vi "Statistics.vi"(0 "image in":refnum<class "MSC Image.lvclass">, 1 "mask image in":refnum<class "MSC Image.lvclass">, 5 "error in (no error)":errorcluster) -> (8 "mean":dbl, 10 "stdDev":dbl, 12 "area":dbl, 14 "image out":refnum<class "MSC Image.lvclass">, 15 "mask image out":refnum<class "MSC Image.lvclass">, 16 "min":dbl, 17 "max":dbl, 19 "error out":errorcluster)   [LabVIEW 2016, in "MSC Image.lvclass"]
doc: "Calculates statistical values of an image with optional mask.\n\nThe image type double can lead to overflows."
uses:
  MSC Image.lvclass
  Dependencies/x86/MSC I Process32.dll
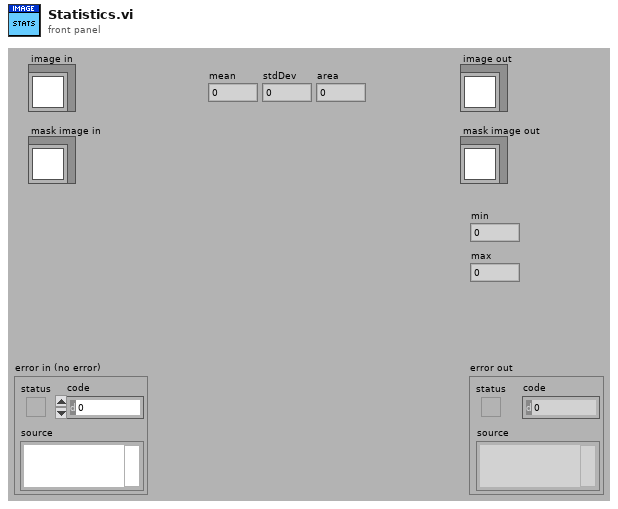
[diagram p1: front panel]
types:
  T1 = typedef "Image.ctl" = cluster{"Pointer":u64, "Size":T2, "Image Type":T3, "Time Stamp":timestamp, "Variant":variant}
  T2 = typedef "Size.ctl" = cluster{"Cols":i32, "Rows":i32}
  T3 = typedef "Image Type.ctl" = i32
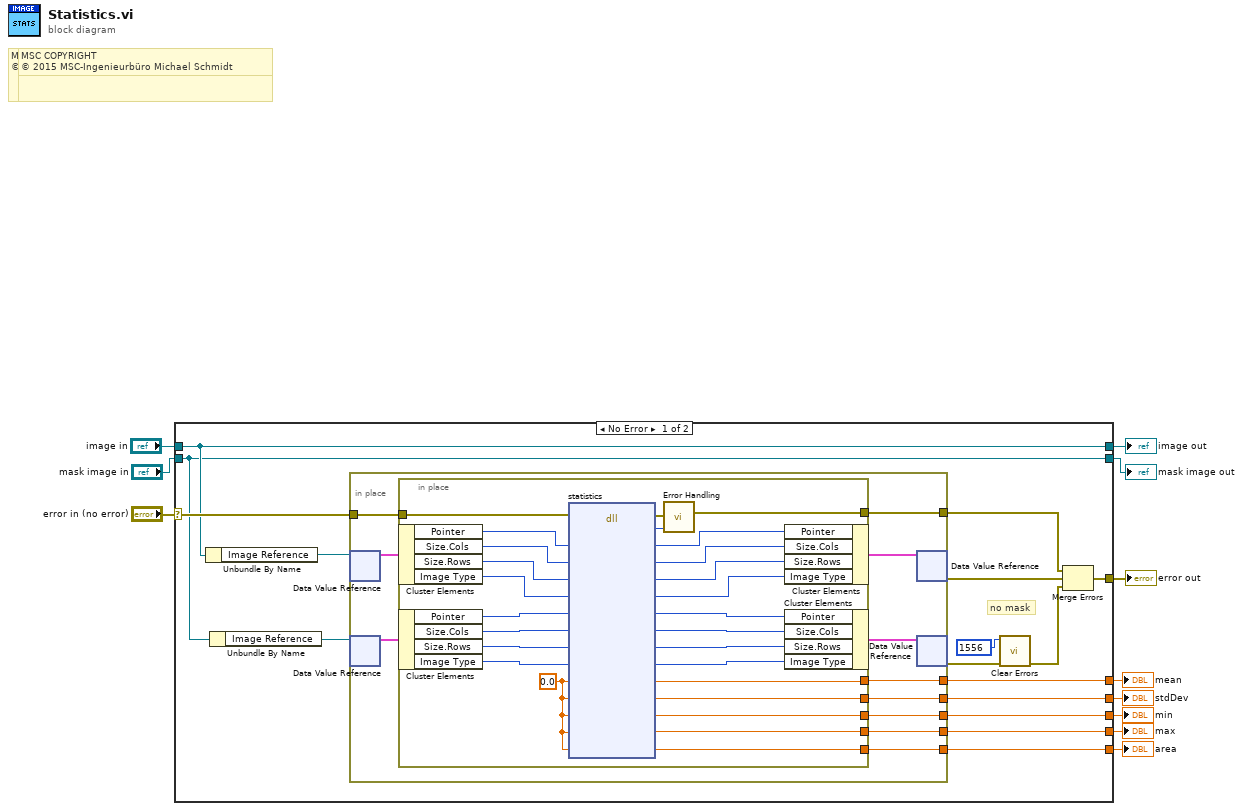
[diagram p0: block diagram]
diagram:
  # "MSC COPYRIGHT\n© 2016 MSC-Ingenieurbüro Michael Schmidt"
  # "MSC COPYRIGHT\n© 2016 MSC-Ingenieurbüro Michael Schmidt"
  # "MSC COPYRIGHT\n© 2015 MSC-Ingenieurbüro Michael Schmidt"
  # "MSC COPYRIGHT\n© 2015 MSC-Ingenieurbüro Michael Schmidt"
  n1 = case shown="No Error" "error in (no error)" {
    selector: "error in (no error)" -> [w16 w67]
    tunnel: [w27 w67] -> w6
    tunnel: [w12 w65] -> w8
    tunnel: "image in" -> [w15 w66]
    tunnel: "mask image in" -> [w12 w65]
    tunnel: [w15 w66] -> w11
    tunnel: [w21 _] -> w5
    tunnel: [w20 _] -> w4
    tunnel: [w24 _] -> w3
    tunnel: [w23 _] -> w2
    tunnel: [w22 _] -> w1
    frame No Error {
      # "no mask"
      n2 = Unbundle By Name(w15) -> ("Image Reference"=w14:refnum<data-value>)
      n3 = Unbundle By Name(w12) -> ("Image Reference"=w13:refnum<data-value>)
      n4 = in-place {
        in-place-border: w16 -> [w36]
        in-place-border: [w35] -> w26
        in-place-border: [w32] -> w21
        in-place-border: [w31] -> w20
        in-place-border: [w30] -> w24
        in-place-border: [w29] -> w23
        in-place-border: [w28] -> w22
        n5 = in-place-dvr #1(w14) -> (w37:T1)  [unwired: 1 out]
        n6 = in-place-dvr #2(w13) -> (w34:T1)  [unwired: 1 out]
        n7 = in-place {
          in-place-border: w36 -> [w39]
          in-place-border: [w50] -> w35
          in-place-border: [w64] -> w32
          in-place-border: [w63] -> w31
          in-place-border: [w62] -> w30
          in-place-border: [w61] -> w29
          in-place-border: [w60] -> w28
          w48 = 0.0 ("mean")
          n8 = in-place-cluster #3(w37) -> ("Pointer"=w47:u64, "Size.Cols"=w46:i32, "Size.Rows"=w45:i32, "Image Type"=w44:T3)
          n9 = in-place-cluster #4(w34) -> ("Pointer"=w43:u64, "Size.Cols"=w42:i32, "Size.Rows"=w41:i32, "Image Type"=w40:T3)
          n10 = dll-call lib="C:/Users/MSC/LabVIEW Projekte/LV 2014/MSC I-Process/user.lib/MSC-I Process/Dependencies/x86/MSC I Process*.dll" fn="statistics"(error in=w39, "pointer"=w47, "cols"=w46, "rows"=w45, "type"=w44, "pointerMask"=w43, "colsMask"=w42, "rowsMask"=w41, "typeMask"=w40, "mean"=w48, "stdDev"=w48, "min"=w48, "max"=w48, "area"=w48) -> (error out=w52:errorcluster, "error"=w51:i32, "pointer"=w49:u64, "cols"=w53:i32, "rows"=w54:i32, "type"=w55:i32, "pointerMask"=w59:u64, "colsMask"=w58:i32, "rowsMask"=w57:i32, "typeMask"=w56:i32, "mean"=w64:dbl, "stdDev"=w63:dbl, "min"=w62:dbl, "max"=w61:dbl, "area"=w60:dbl)  [unwired: 2 in, 1 out]
          n11 = call "Error Handling.vi"("error in (no error)"=w52, "return type"=w51) -> ("error out"=w50:errorcluster)  [unwired: 12 in, 1 out]
          n12 = in-place-cluster #3("Pointer"=w49, "Size.Cols"=w53, "Size.Rows"=w54, "Image Type"=w55) -> (w38:T1)
          n13 = in-place-cluster #4("Pointer"=w59, "Size.Cols"=w58, "Size.Rows"=w57, "Image Type"=w56) -> (w33:T1)
        }
        n14 = in-place-dvr #1(w38) -> (w25:errorcluster)  [unwired: 1 out]
        n15 = in-place-dvr #2(w33) -> (w18:errorcluster)  [unwired: 1 out]
      }
      n16 = call <vilib>:"Clear Errors.vi"("error in (no error)"=w18, "specific error code to clear (0: all)"=1556) -> ("error out"=w19:errorcluster)  [unwired: 4 in, 1 out]
      n17 = Merge Errors(w26, w25, w19) -> (w27:errorcluster)
    }
    frame Error {
    }
  }
  "error out" <- w6
  "image out" <- w11
  "mask image out" <- w8
  "mean" <- w5
  "stdDev" <- w4
  "min" <- w3
  "max" <- w2
  "area" <- w1
